vi "Apply_Container_Settings.vi"(8 "error in (no error)":errorcluster, 11 "AB_Build in":refnum<class "AB_Build.lvclass">) -> (0 "error out":errorcluster, 3 "AB_Build out":refnum<class "AB_Build.lvclass">)   [LabVIEW 2020, in "AB_Build.lvclass"]
uses:
  <vilib>/AppBuilder/AB_Classes/Build/AB_Build.lvclass
  <vilib>/AppBuilder/AB_Classes/Build/AB_Build.lvclass/AB_Build.ctl
  <vilib>/AppBuilder/AB_Classes/Source/AB_Source.lvclass
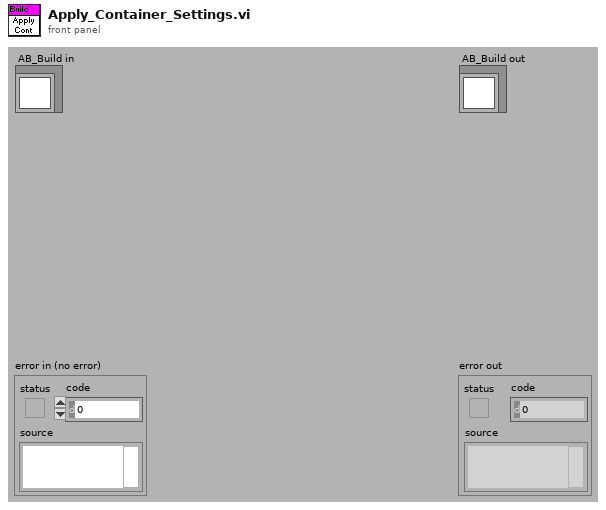
[diagram p1: front panel]
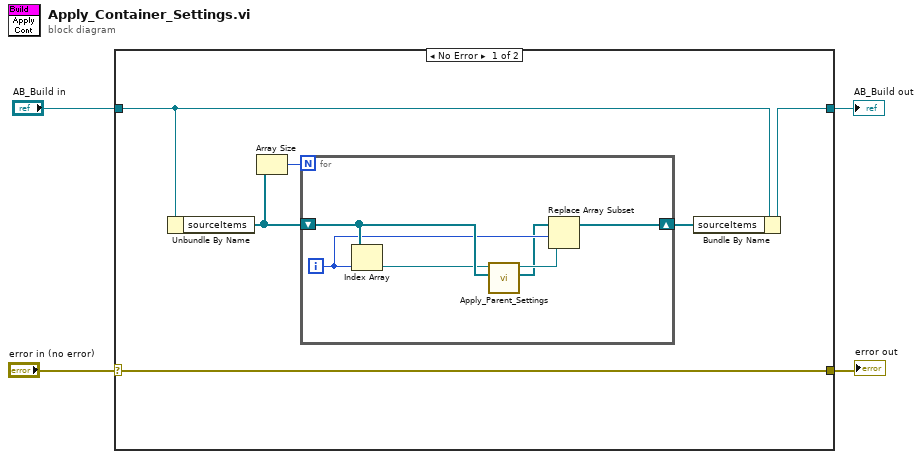
[diagram p0: block diagram]
diagram:
  n1 = case shown="No Error" "error in (no error)" {
    selector: "error in (no error)" -> [w10 w18]
    tunnel: [w10 w18] -> w3
    tunnel: [w5 w17] -> w1
    tunnel: "AB_Build in" -> [w6 w17]
    frame No Error {
      n2 = Unbundle By Name(w6) -> ("sourceItems"=w8:refnum<class "AB_Source.lvclass">[])
      n3 = Array Size(array=w8) -> (size(s)=w9:i32)
      n4 = for {
        N: w9 -> [_]
        shift-right: [w16] -> w7
        shift-left: w8 -> [w15]
        i -> [w14]
        n5 = Index Array(array=w15, index=w14) -> (element=w13:refnum<class "AB_Source.lvclass">)
        n6 = call-dynamic "Apply_Parent_Settings.vi"("sourceItems in"=w15, "AB_Source in"=w13) -> ("sourceItems out"=w11:refnum<class "AB_Source.lvclass">[], "AB_Source out"=w12:refnum<class "AB_Source.lvclass">)  [unwired: 6 in, 2 out]
        n7 = Replace Array Subset(array=w11, new element=w12, index=w14) -> (w16:refnum<class "AB_Source.lvclass">[])
      }
      n8 = Bundle By Name(cluster=w6, "sourceItems"=w7) -> (w5:refnum<class "AB_Build.lvclass">)
    }
    frame Error {
    }
  }
  "error out" <- w3
  "AB_Build out" <- w1
